vi "MH_BufferRecord.vi"(6 "WindowWidth":i32, 7 "truetime":u64, 8 "WinIndex":i32, 9 "Buffindex":i32, 10 "Buffsize":i32, 11 "Buffer":u64[](array[numeric])) -> (0 "WinIndexOut":i32, 1 "BuffIndexOut":i32, 2 "NewBuffsize":i32, 3 "tableau (n rotations)":u64[](array[numeric]))   [LabVIEW 2019]
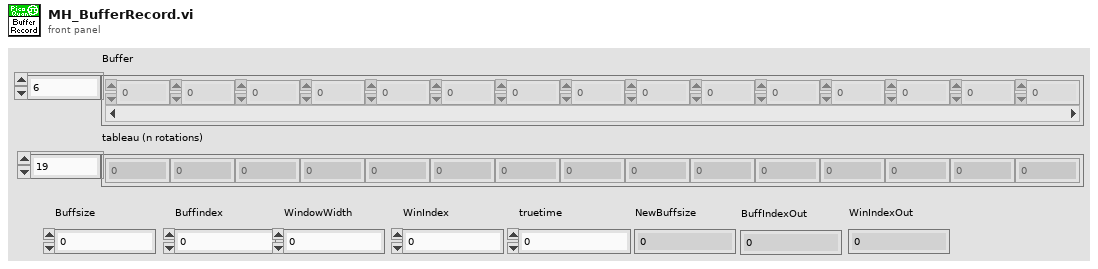
[diagram p1: front panel]
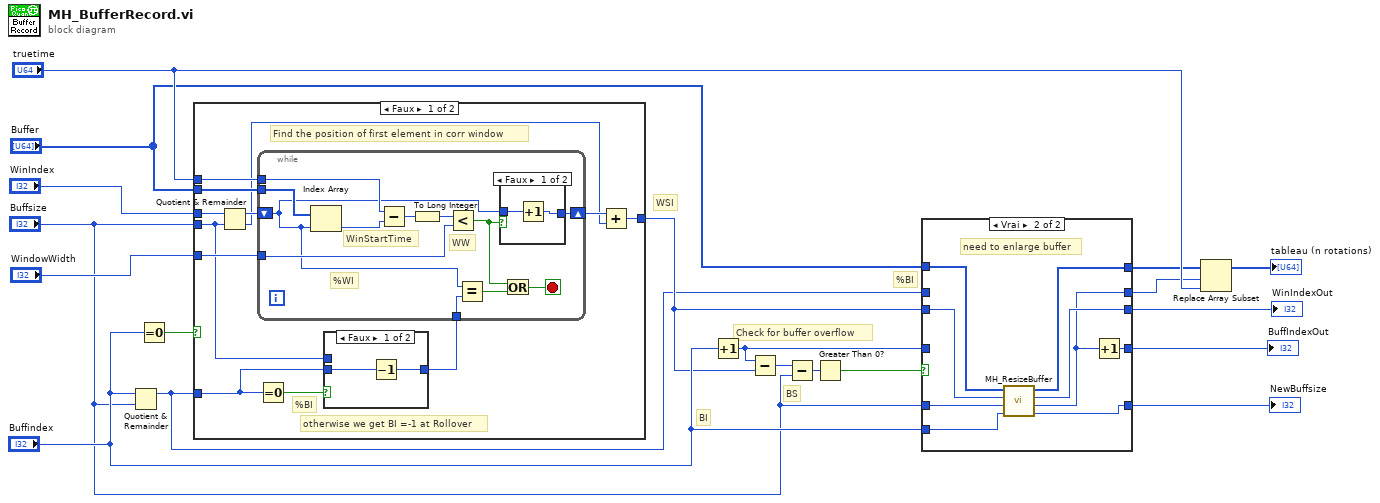
[diagram p0: block diagram]
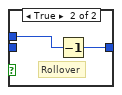
[diagram p3: hidden frame]
diagram:
  # "%BI"
  # "BS"
  # "Check for buffer overflow"
  # "WSI"
  # "BI"
  n1 = Quotient & Remainder(x="Buffindex", y="Buffsize") -> (x-y*floor(x/y)=w2:i32)  [unwired: 1 out]
  n2 = Equal To 0?(x="Buffindex") -> (x = 0?=w5:bool)
  n3 = case shown="Faux" w5 {
    tunnel: "truetime" -> [w31 _]
    tunnel: "WinIndex" -> [w21 w51]
    tunnel: "WindowWidth" -> [w30 _]
    tunnel: "Buffer" -> [w29 _]
    tunnel: [w22 w51] -> w7
    tunnel: "Buffsize" -> [w24 _]
    tunnel: w2 -> [w27 _]
    frame False {
      # "Find the position of first element in corr window"
      # "otherwise we get BI =-1 at Rollover"
      # "%BI"
      n4 = Quotient & Remainder(x=w21, y=w24) -> (x-y*floor(x/y)=w23:i32, floor(x/y)=w20:i32)
      n5 = Equal To 0?(x=w27) -> (x = 0?=w25:bool)
      n6 = case shown="Faux" w25 {
        tunnel: w27 -> [w48 _]
        tunnel: [w47 w49] -> w26
        tunnel: w24 -> [_ w50]
        frame False {
          n7 = Decrement(x=w48) -> (x-1=w47:i32)
        }
        frame True {
          # "Rollover"
          n8 = Decrement(x=w50) -> (x-1=w49:i32)
        }
      }
      n9 = while {
        tunnel: w31 -> [w43]
        tunnel: w29 -> [w42]
        shift-right: [w35] -> w28
        shift-left: w23 -> [w32]
        tunnel: w30 -> [w39]
        tunnel: w26 -> [w36]
        stop <- w37 stop-if-true
        # "WW"
        # "%WI"
        # "WinStartTime"
        n10 = Index Array(array=w42, index=w32) -> (element=w41:u64)
        n11 = Subtract(x=w43, y=w41) -> (x-y=w40:u64)
        n12 = To Long Integer(number=w40) -> (32bit integer=w38:i32)
        n13 = Less?(x=w38, y=w39) -> (x < y?=w33:bool)
        n14 = Equal?(x=w32, y=w36) -> (x = y?=w34:bool)
        n15 = case shown="Faux" w33 {
          tunnel: w32 -> [w45 w46]
          tunnel: [w44 w46] -> w35
          frame False {
            n16 = Increment(x=w45) -> (x+1=w44:i32)
          }
          frame True {
          }
        }
        n17 = Or(x=w33, y=w34) -> (x .or. y?=w37:bool)
      }
      n18 = Add(x=w28, y=w20) -> (x+y=w22:i32)
    }
    frame True {
      # "no need to check WSI"
      # "BufferIndex = 0"
    }
  }
  n19 = Increment(x="Buffindex") -> (x+1=w4:i32)
  n20 = Subtract(x=w4, y=w7) -> (x-y=w11:i32)
  n21 = Subtract(x=w11, y="Buffsize") -> (x-y=w10:i32)
  n22 = Greater Than 0?(x=w10) -> (x > 0?=w8:bool)
  n23 = case shown="Vrai" w8 {
    tunnel: "Buffer" -> [w54 w65]
    tunnel: "Buffsize" -> [w55 w62]
    tunnel: [w54 w64] -> w9
    tunnel: "Buffindex" -> [_ w63]
    tunnel: w7 -> [w56 w61]
    tunnel: [w53 w58] -> w6
    tunnel: [w56 w60] -> w12
    tunnel: w2 -> [w53 _]
    tunnel: w4 -> [w52 _]
    tunnel: [w55 w59] -> w3
    tunnel: [w52 w57] -> w1
    frame False {
    }
    frame True {
      # "need to enlarge buffer"
      n24 = call <userlib>:"MH_ResizeBuffer.vi"("Buffindex"=w63, "Buffsize"=w62, "WinIndex"=w61, "Tableau"=w65) -> ("NewBuffsize"=w59:i32, "NewBuffIndex"=w58:i32, "NewWinIndex"=w60:i32, "tableau (n rotations)"=w64:u64[])  [unwired: 2 in, 2 out]
      n25 = Increment(x=w58) -> (x+1=w57:i32)
    }
  }
  "BuffIndexOut" <- w1
  "WinIndexOut" <- w12
  "NewBuffsize" <- w3
  n26 = Replace Array Subset(array=w9, new element="truetime", index=w6) -> (→"tableau (n rotations)":u64[])
